vi "Flatten XML.vi"(8 "Error In":errorcluster, 9 "Save UIP List (True)":bool=TRUE, 11 "UIM In":refnum<data-value>) -> (0 "Error Out":errorcluster, 2 "XML":string, 3 "UIM Out":refnum<data-value>)   [LabVIEW 2015, in "UIM.lvclass"]
doc: "This method will convert the UIM data into XML format that is easy to read. The same format is used when the UIM is saved and loaded to and from XML file."
uses:
  UIM.lvclass
  <vilib>/xml/Close Reference(Node).vi
  <vilib>/xml/NI_XML.lvlib
  <resource>/objmgr/DOMUserDefRef.rc
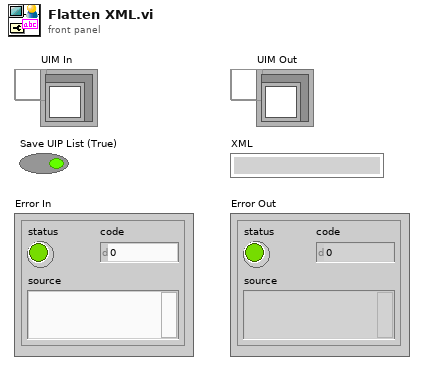
[diagram p1: front panel]
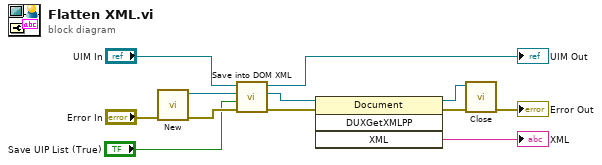
[diagram p0: block diagram]
diagram:
  n1 = call <vilib>:"New.vi"("error in (no error)"="Error In") -> ("error out"=w8:errorcluster, "DOM document out"=w5:refnum<k20>)  [unwired: 7 in]
  n2 = call "Save into DOM XML.vi"("Error In"=w8, "Save UIP List (True)"="Save UIP List (True)", "DOM In"=w5, "UIM In"="UIM In") -> ("Error Out"=w4:errorcluster, "DOM Out"=w3:refnum<k20>, "UIM Out"=→"UIM Out":refnum<data-value>)  [unwired: 5 in]
  n3 = invoke class="Document" method="DUXGetXMLPP"(reference=w3, error in=w4) -> (reference out=w11:refnum<k20>, error out=w12:errorcluster, "XML"=→"XML":string)  [unwired: 2 in, 1 out]
  n4 = call-poly <vilib>:"Close.vi"("error in (no error)"=w12, "node"=w11) -> ("error out"=→"Error Out":errorcluster)  [unwired: 7 in]
